vi "數位濾波+數位積分版V4.vi"() -> ()   [LabVIEW 2010]
uses:
  <vilib>/Analysis/3filter.llb/Filter Passband Type.ctl
  <vilib>/DAQmx/read.llb/DAQmx Read (Analog DBL 1Chan 1Samp).vi
  <vilib>/DAQmx/write.llb/DAQmx Write (Analog DBL 1Chan 1Samp).vi
  <vilib>/DAQmx/create/channels.llb/DAQmx Create Channel (AI-Voltage-Basic).vi
  <vilib>/DAQmx/configure/timing.llb/DAQmx Timing (Sample Clock).vi
  <vilib>/DAQmx/create/channels.llb/DAQmx Create Channel (AO-Voltage-Basic).vi
  <vilib>/daqmx/miscellaneous.llb/DAQmx Fill In Error Info.vi
  <vilib>/Analysis/3filter.llb/Butterworth Filter (DBL).vi
  <vilib>/Analysis/NI_AALBase.lvlib
panel:
  in  "輸入訊號縮放比例":dbl=1.0
  in  "ÂoDC?":bool
  in  "Kv":dbl=-5000.0
  in  "濾波階數":i32=2
  in  "low cutoff freq":dbl=50.0 format="%0.4f"
  in  "濾波?":bool
  out "理想迴圈時間":dbl
  out "延遲警告":bool
  out "當下DC值":dbl
  in  "DAQ input":tag
  in  "DAQ output":tag
  in  "Ka":dbl=-300.0
  out "message":string=" INSTRUCTIONS:\r\rNormal Use:  When using subVIs that incorporate the error in/error out (or error I/O) structure, place this handler where you want to inform the user of an error, typically at the end of the I/O data path, as the last action of the program.  If the error in error? is ERROR, the handler creates a message describing the error and its source.  If the type of dialog = 1 (default), the message is displayed to the user, who can only acknowedge it.  If the type = 2, the user can acknowledge the message or abort execution; aborting a program with active I/O is not recommended.  If the type = 0, no message is displayed; this is used to process the error programmatically, and the error out cluster elements are wired to individual terminals for that reason.  \r\rOther Use:\n\r\nlocal testing.  To test the error code of a subVI or function that does not have the error I/O structure, you can wire its error code and a source string to the local error code and error source inputs.  If error in error? indicates no error and error code is not equal to 0, the local code and source are substituted for the error in values, and error? is set TRUE (ERROR)."
  out "while平均運行時間":dbl
  in  "取樣頻率":dbl=5000.0 min=1.0 max=20000.0 step=1.0
  in  "stop":bool
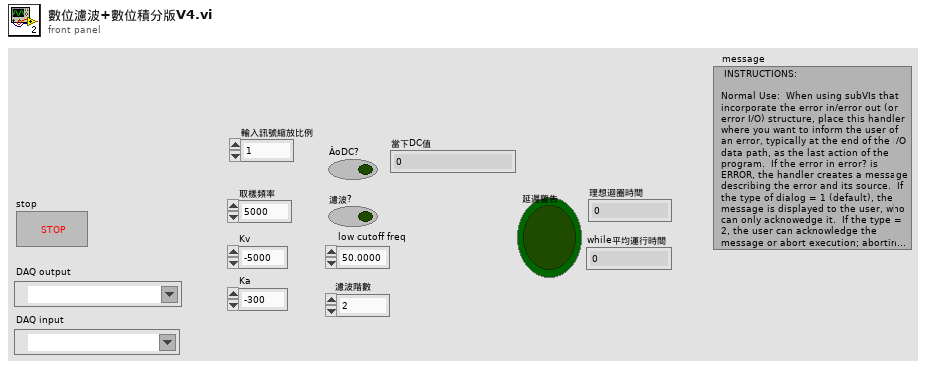
[diagram p1: front panel]
types:
  T1 = typedef "NI_AALBase.lvlib/Filter Passband Type.ctl" = enum32{"Lowpass", "Highpass", "Bandpass", "Bandstop"}
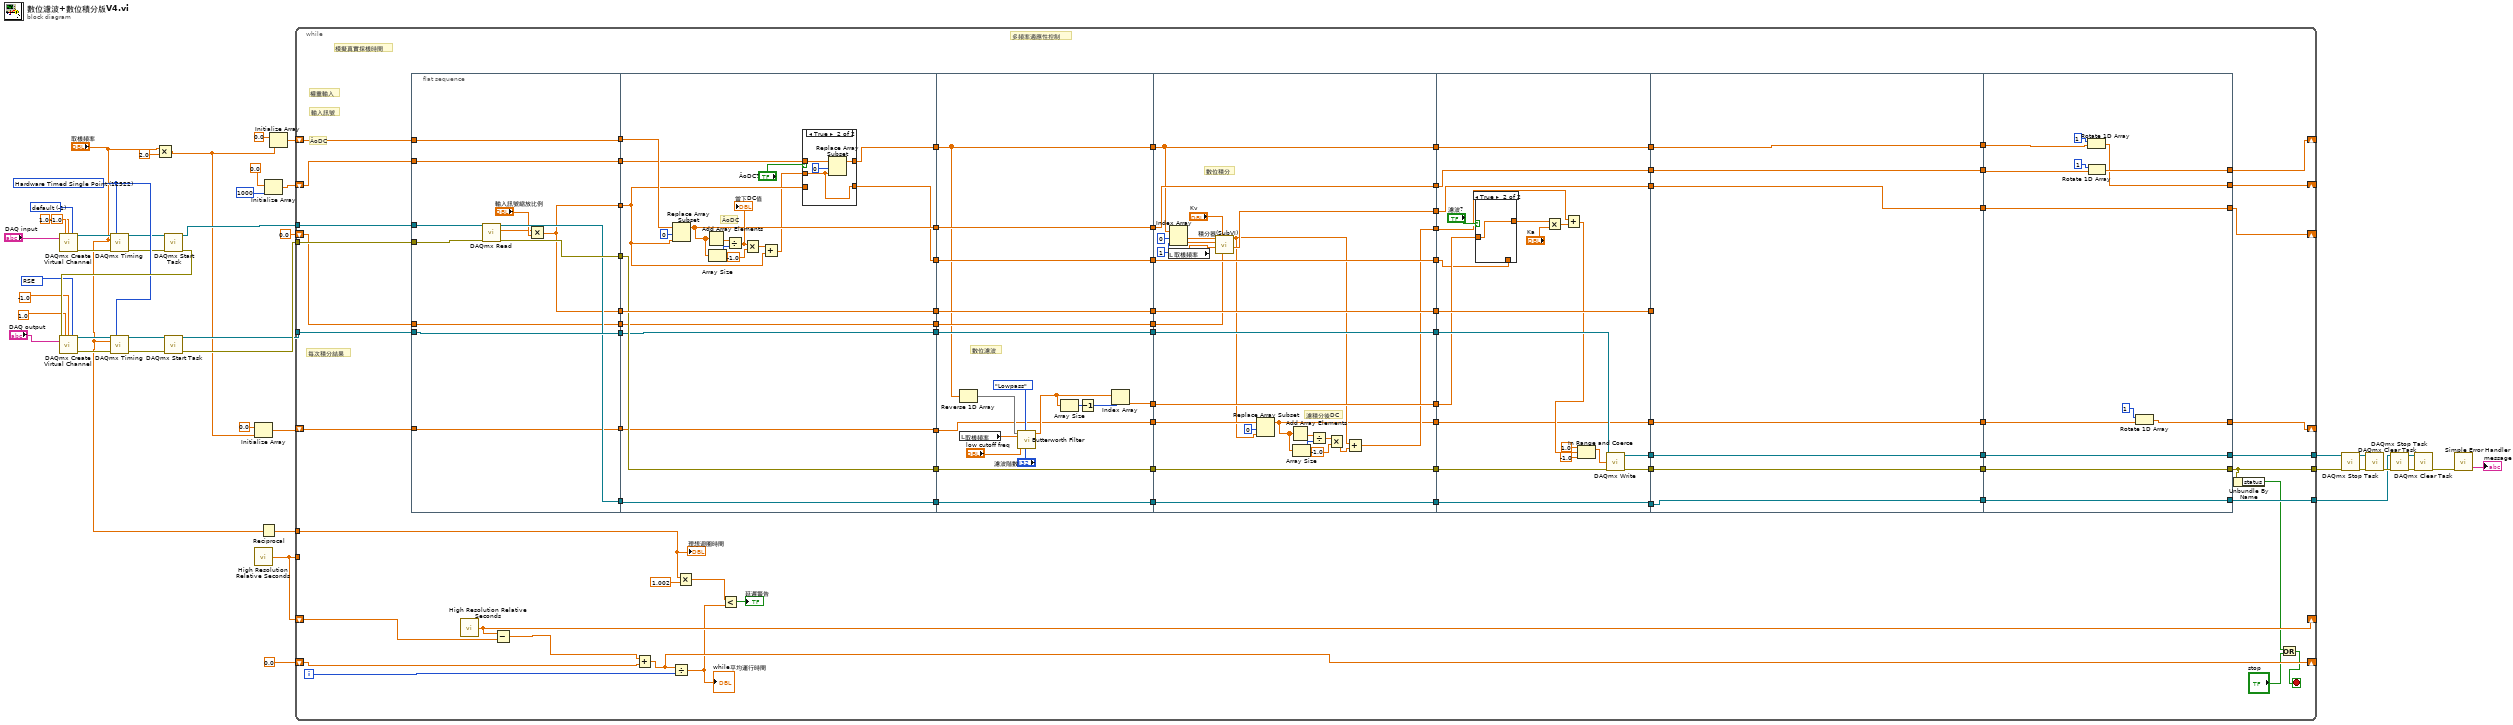
[diagram p0: block diagram]
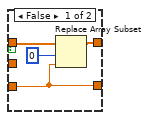
[diagram p2: hidden frame]
diagram:
  w39 = 12522 items=["Finite Samples"=10178, "Continuous Samples"=10123, "Hardware Timed Single Point"=12522] ("sample mode")
  w36 = 10083 items=["Default"=-1, "RSE"=10083, "Differential"=10106, "Pseudodifferential"=12529] ("output terminal configuration")
  w35 = -1 items=["default"=-1, "RSE"=10083, "NRSE"=10078, "Differential"=10106, "Pseudodifferential"=12529] ("input terminal configuration")
  n1 = call-poly <vilib>:"DAQmx Create Virtual Channel.vi"("maximum value"=1.0, "minimum value"=-1.0, "input terminal configuration"=w35, "physical channels"="DAQ input") -> ("task out"=w27:refnum<k21>, "error out"=w30:errorcluster)  [unwired: 10 in]
  n2 = call-poly <vilib>:"DAQmx Timing.vi"("task/channels in"=w27, "sample mode"=w39, "rate"="取樣頻率", "error in"=w30) -> ("task out"=w28:refnum<k21>, "error out"=w29:errorcluster)  [unwired: 10 in]
  n3 = Multiply(x="取樣頻率", y=2.0) -> (x*y=w1:dbl)
  n4 = call <vilib>:"DAQmx Start Task.vi"("task/channels in"=w28, "error in"=w29) -> ("task out"=w7:refnum<k21>, "error out"=w42:errorcluster)  [unwired: 12 in]
  n5 = call-poly <vilib>:"DAQmx Create Virtual Channel.vi"("maximum value"=1.0, "minimum value"=-1.0, "output terminal configuration"=w36, "physical channels"="DAQ output", "error in"=w42) -> ("task out"=w34:refnum<k21>, "error out"=w31:errorcluster)  [unwired: 9 in]
  n6 = call-poly <vilib>:"DAQmx Timing.vi"("task/channels in"=w34, "sample mode"=w39, "rate"="取樣頻率", "error in"=w31) -> ("task out"=w33:refnum<k21>, "error out"=w32:errorcluster)  [unwired: 10 in]
  n7 = call <vilib>:"DAQmx Start Task.vi"("task/channels in"=w33, "error in"=w32) -> ("task out"=w25:refnum<k21>, "error out"=w26:errorcluster)  [unwired: 12 in]
  n8 = Initialize Array(0.0 ("element"), w1) -> (w5:dbl[])
  n9 = call <vilib>:"High Resolution Relative Seconds.vi"() -> ("relative seconds"=w45:dbl)
  n10 = Reciprocal(x="取樣頻率") -> (1/x=w10:dbl)
  n11 = Initialize Array(0.0 ("element"), 1000 ("dimension size")) -> (w11:dbl[])
  n12 = Initialize Array(0.0 ("element"), w1) -> (w13:dbl[])
  n13 = while {
    tunnel: w45 -> [_]
    shift-right: [w123] -> _
    shift-left: w45 -> [w122]
    shift-right: [w124] -> _
    shift-left: 0.0 -> [w126]
    shift-right: [w116] -> _
    shift-left: w13 -> [w118]
    tunnel: w7 -> [w113]
    tunnel: w26 -> [w112]
    tunnel: w25 -> [w111]
    tunnel: [w107] -> w19
    tunnel: [w98] -> w18
    tunnel: [w101] -> w17
    shift-right: [w85] -> _
    shift-left: w11 -> [w89]
    tunnel: w10 -> [w82]
    shift-right: [w72] -> _
    shift-left: 0.0 ("輸出累加ERR回朔") -> [w77]
    shift-right: [w49] -> _
    shift-left: w5 -> [w53]
    i -> [w125]
    stop <- w100 stop-if-true
    # "每次積分結果"
    # "權重輸入"
    # "輸入訊號"
    # "ÂoDC"
    # "模擬真實採樣時間"
    # "多頻率適應性控制"
    n14 = flat-sequence {
      tunnel: [w129] -> w127
      tunnel: [w129] -> w120
      tunnel: [w136] -> w119
      tunnel: w118 -> [w139]
      tunnel: [w139] -> w117
      tunnel: w113 -> [w138]
      tunnel: w112 -> [w137]
      tunnel: w111 -> [w135]
      tunnel: [w135] -> w110
      tunnel: [w134] -> w104
      tunnel: [w133] -> w90
      tunnel: w89 -> [w133]
      tunnel: w77 -> [w132]
      tunnel: [w132] -> w76
      tunnel: [w131] -> w54
      tunnel: w53 -> [w131]
      tunnel: w127 -> [w142]
      tunnel: [w158] -> w71
      tunnel: [w159] -> w69
      tunnel: w120 -> [w159]
      tunnel: w119 -> [w158]
      tunnel: w117 -> [w156]
      tunnel: [w143] -> w67
      tunnel: [w150] -> w65
      tunnel: w110 -> [w150]
      tunnel: [w149] -> w63
      tunnel: w104 -> [w149]
      tunnel: w90 -> [w148]
      tunnel: [w147] -> w61
      tunnel: w76 -> [w145]
      tunnel: [w146] -> w58
      tunnel: [w145] -> w56
      tunnel: w54 -> [w140]
      tunnel: [w140] -> w52
      tunnel: w71 -> [w185]
      tunnel: [w185] -> w70
      tunnel: w69 -> [w184]
      tunnel: [w184] -> w68
      tunnel: w67 -> [w183]
      tunnel: [w183] -> w66
      tunnel: w65 -> [w182]
      tunnel: [w182] -> w64
      tunnel: w63 -> [w181]
      tunnel: [w181] -> w62
      tunnel: w61 -> [w169]
      tunnel: [w169] -> w60
      tunnel: [w170] -> w59
      tunnel: w58 -> [w180]
      tunnel: [w180] -> w57
      tunnel: w56 -> [w179]
      tunnel: [w179] -> w55
      tunnel: w52 -> [w168]
      tunnel: [w168] -> w51
      tunnel: w70 -> [w211]
      tunnel: [w211] -> w96
      tunnel: w68 -> [w210]
      tunnel: [w210] -> w95
      tunnel: [w200] -> w94
      tunnel: w66 -> [w209]
      tunnel: [w209] -> w93
      tunnel: w64 -> [w208]
      tunnel: [w208] -> w92
      tunnel: w62 -> [w207]
      tunnel: [w207] -> w91
      tunnel: [w197] -> w86
      tunnel: w60 -> [w197]
      tunnel: w59 -> [w206]
      tunnel: [w206] -> w84
      tunnel: w57 -> [w200]
      tunnel: [w196] -> w74
      tunnel: w55 -> [w201]
      tunnel: w51 -> [w190]
      tunnel: [w187] -> w50
      tunnel: [w186] -> w46
      tunnel: w96 -> [w229]
      tunnel: [w221] -> w121
      tunnel: w95 -> [w221]
      tunnel: [w231] -> w114
      tunnel: w94 -> [w231]
      tunnel: w93 -> [w217]
      tunnel: w92 -> [w230]
      tunnel: [w228] -> w108
      tunnel: [w227] -> w106
      tunnel: w91 -> [w226]
      tunnel: [w226] -> w103
      tunnel: [w222] -> w87
      tunnel: w86 -> [w222]
      tunnel: w84 -> [w219]
      tunnel: [w216] -> w75
      tunnel: w74 -> [w216]
      tunnel: w50 -> [w214]
      tunnel: [w212] -> w47
      tunnel: w46 -> [w212]
      tunnel: w121 -> [_]
      tunnel: [w238] -> w115
      tunnel: w114 -> [w238]
      tunnel: [w241] -> w109
      tunnel: w108 -> [w241]
      tunnel: w106 -> [w240]
      tunnel: [w240] -> w105
      tunnel: w103 -> [w239]
      tunnel: [w239] -> w102
      tunnel: [w237] -> w88
      tunnel: w87 -> [w237]
      tunnel: w75 -> [w236]
      tunnel: [w236] -> w73
      tunnel: [w235] -> w48
      tunnel: w47 -> [w235]
      tunnel: [w253] -> w116
      tunnel: w115 -> [w252]
      tunnel: w109 -> [w251]
      tunnel: [w251] -> w107
      tunnel: [w250] -> w98
      tunnel: w105 -> [w250]
      tunnel: w102 -> [w249]
      tunnel: [w249] -> w101
      tunnel: w88 -> [w247]
      tunnel: [w246] -> w85
      tunnel: [w245] -> w72
      tunnel: w73 -> [w245]
      tunnel: [w242] -> w49
      tunnel: w48 -> [w243]
      frame #0 {
        n15 = call-poly <vilib>:"DAQmx Read.vi"("task/channels in"=w138, "error in"=w137) -> ("task out"=w134:refnum<k21>, "data"=w128:dbl, "error out"=w136:errorcluster)  [unwired: 11 in]
        n16 = Multiply(x=w128, y="輸入訊號縮放比例") -> (x*y=w129:dbl)
      }
      frame #1 {
        # "ÂoDC"
        n17 = Replace Array Subset(array=w156, new element=w142, index=0) -> (w146:dbl[])
        n18 = Add Array Elements(numeric array=w146) -> (sum=w155:dbl)
        n19 = Array Size(array=w146) -> (size(s)=w154:i32)
        n20 = Divide(x=w155, y=w154) -> (x/y=w153:dbl)
        "當下DC值" <- w153
        n21 = Multiply(x=w153, y=-1.0) -> (x*y=w151:dbl)
        n22 = Add(x=w151, y=w142) -> (x+y=w141:dbl)
        n23 = case shown="True" "ÂoDC?" {
          tunnel: w148 -> [w161 w166]
          tunnel: [w162 w165] -> w147
          tunnel: w141 -> [_ w164]
          tunnel: w142 -> [w160 _]
          tunnel: [w160 w164] -> w143
          frame False {
            n24 = Replace Array Subset(array=w161, new element=w160, index=0) -> (w162:dbl[])
          }
          frame True {
            n25 = Replace Array Subset(array=w166, new element=w164, index=0) -> (w165:dbl[])
          }
        }
      }
      frame #2 {
        # "數位濾波"
        n26 = Reverse 1D Array(array=w169) -> (reversed array=w173:dbl[])
        n27 = local read "取樣頻率"() -> (w171:dbl)
        n28 = call-poly <vilib>:"Butterworth Filter.vi"("order"="濾波階數", "filter type"=Filter_Passband_Type."Lowpass", "low cutoff freq: fl"="low cutoff freq", "sampling freq: fs"=w171, "X"=w173) -> ("Filtered X"=w174:dbl[])  [unwired: 3 in, 1 out]
        n29 = Array Size(array=w174) -> (size(s)=w175:i32)
        n30 = Decrement(x=w175) -> (x-1=w176:i32)
        n31 = Index Array(array=w174, index=w176) -> (element=w170:dbl)
      }
      frame #3 {
        # "濾積分後DC"
        # "數位積分"
        n32 = local read "取樣頻率"() -> (w199:dbl)
        n33 = Index Array(array=w197, index #1=0 ("index"), index #2=1 ("index")) -> (element #1=w203:dbl, element #2=w202:dbl)
        n34 = call "積分器(SubVI).vi"("輸入累加ERR回朔"=w201, "I增益"="Kv", "samples (Hz)"=w199, "前一個ERR"=w202, "當下ERR"=w203) -> ("輸出累加ERR回朔"=w196:dbl, "積分修正量"=w189:dbl)  [unwired: 5 in]
        n35 = Replace Array Subset(array=w190, new element=w189, index=0) -> (w186:dbl[])
        n36 = Add Array Elements(numeric array=w186) -> (sum=w194:dbl)
        n37 = Array Size(array=w186) -> (size(s)=w193:i32)
        n38 = Divide(x=w194, y=w193) -> (x/y=w192:dbl)
        n39 = Multiply(x=w192, y=-1.0) -> (x*y=w188:dbl)
        n40 = Add(x=w189, y=w188) -> (x+y=w187:dbl)
      }
      frame #4 {
        n41 = case shown="True" "濾波?" {
          tunnel: w219 -> [_ w234]
          tunnel: [w233 w234] -> w218
          tunnel: w217 -> [w233 _]
          frame False {
          }
          frame True {
          }
        }
        n42 = Multiply(x=w218, y="Ka") -> (x*y=w215:dbl)
        n43 = Add(x=w214, y=w215) -> (x+y=w213:dbl)
        n44 = In Range and Coerce(upper limit=1.0, x=w213, lower limit=-1.0) -> (coerced(x)=w225:dbl)  [unwired: 1 out]
        n45 = call-poly <vilib>:"DAQmx Write.vi"("task/channels in"=w230, "data"=w225, "error in"=w229) -> ("task out"=w228:refnum<k21>, "error out"=w227:errorcluster)  [unwired: 10 in, 1 out]
      }
      frame #5 {
      }
      frame #6 {
        n46 = Rotate 1D Array(1:w247, 2:1 ("n")) -> (0:w246:dbl[])
        n47 = Rotate 1D Array(1:w252, 2:1 ("n")) -> (0:w253:dbl[])
        n48 = Rotate 1D Array(1:w243, 2:1 ("n")) -> (0:w242:dbl[])
      }
    }
    n49 = call <vilib>:"High Resolution Relative Seconds.vi"() -> ("relative seconds"=w123:dbl)
    n50 = Subtract(x=w123, y=w122) -> (x-y=w83:dbl)
    n51 = Add(x=w83, y=w126) -> (x+y=w124:dbl)
    n52 = Divide(x=w124, y=w125) -> (x/y=w79:dbl)
    "while平均運行時間" <- w79
    n53 = Multiply(x=w82, y=1.002) -> (x*y=w80:dbl)
    n54 = Less?(x=w80, y=w79) -> (x < y?=→"延遲警告":bool)
    n55 = Unbundle By Name(w98) -> ("status"=w97:bool)
    n56 = Or(x=w97, y="stop") -> (x .or. y?=w100:bool)
    "理想迴圈時間" <- w82
  }
  n57 = call <vilib>:"DAQmx Stop Task.vi"("task/channels in"=w19, "error in"=w18) -> ("task out"=w20:refnum<k21>, "error out"=w21:errorcluster)  [unwired: 12 in]
  n58 = call <vilib>:"DAQmx Clear Task.vi"("task in"=w20, "error in"=w21) -> ("error out"=w24:errorcluster)  [unwired: 13 in]
  n59 = call <vilib>:"DAQmx Stop Task.vi"("task/channels in"=w17, "error in"=w24) -> ("task out"=w23:refnum<k21>, "error out"=w22:errorcluster)  [unwired: 12 in]
  n60 = call <vilib>:"DAQmx Clear Task.vi"("task in"=w23, "error in"=w22) -> ("error out"=w16:errorcluster)  [unwired: 13 in]
  n61 = call <vilib>:"Simple Error Handler.vi"("error in (no error)"=w16) -> ("message"=→"message":string)  [unwired: 4 in, 4 out]
